vi "old_vi_Filestructure.vi"(4 "Discharge filepath":path, 6 "Batteryname":string, 7 "Charge filepath":path, 8 "For loop i":i32, 9 "In for loop":bool, 11 "Starting Cycle":i32) -> (0 "DischargeWaitPath":path, 1 "DischargeCyclePath":path, 2 "ChargeWaitPath":path, 3 "ChargeCyclePath":path, 5 "Cycle Index":i32)   [LabVIEW 2025]
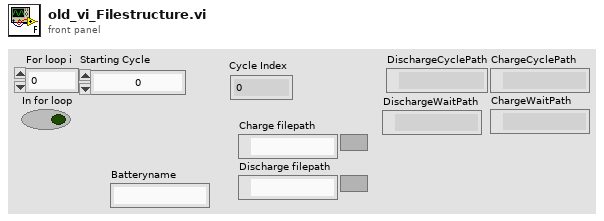
[diagram p1: front panel]
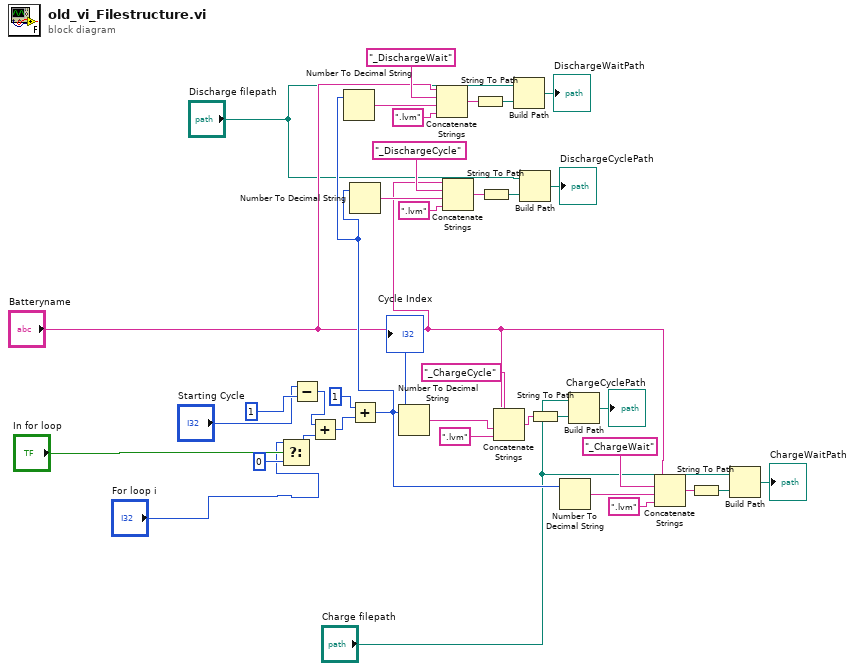
[diagram p0: block diagram]
diagram:
  n1 = Select(t="For loop i", s="In for loop", f=0) -> (s? t:f=w11:i32)
  n2 = Subtract(x="Starting Cycle", y=1) -> (x-y=w8:i32)
  n3 = Add(x=w8, y=w11) -> (x+y=w18:i32)
  n4 = Add(x=1, y=w18) -> (x+y=w19:i32)
  "Cycle Index" <- w19
  n5 = Number To Decimal String(number=w19) -> (decimal integer string=w26:string)  [unwired: 1 in]
  n6 = Number To Decimal String(number=w19) -> (decimal integer string=w31:string)  [unwired: 1 in]
  n7 = Number To Decimal String(number=w19) -> (decimal integer string=w6:string)  [unwired: 1 in]
  n8 = Concatenate Strings("Batteryname", "_DischargeWait", w26, ".lvm") -> (w27:string)
  n9 = Concatenate Strings("Batteryname", "_DischargeCycle", w31, ".lvm") -> (w32:string)
  n10 = String To Path(string=w27) -> (path=w28:path)
  n11 = String To Path(string=w32) -> (path=w33:path)
  n12 = Concatenate Strings("Batteryname", "_ChargeCycle", w6, ".lvm") -> (w35:string)
  n13 = Build Path(base path="Discharge filepath", name or relative path=w28) -> (appended path=→"DischargeWaitPath":path)
  n14 = Build Path(base path="Discharge filepath", name or relative path=w33) -> (appended path=→"DischargeCyclePath":path)
  n15 = String To Path(string=w35) -> (path=w36:path)
  n16 = Number To Decimal String(number=w19) -> (decimal integer string=w21:string)  [unwired: 1 in]
  n17 = Build Path(base path="Charge filepath", name or relative path=w36) -> (appended path=→"ChargeCyclePath":path)
  n18 = Concatenate Strings("Batteryname", "_ChargeWait", w21, ".lvm") -> (w22:string)
  n19 = String To Path(string=w22) -> (path=w23:path)
  n20 = Build Path(base path="Charge filepath", name or relative path=w23) -> (appended path=→"ChargeWaitPath":path)
